vi "Logdata.vi"(7 "Command":T1, 8 "error in (no error)":errorcluster, 10 "Zone Setup Array":cluster{"Zone Selector":string, "Timing":dbl}[](array[cluster]), 11 "file path (dialog if empty)":path) -> (0 "error out":errorcluster, 2 "Zone Setup Array":cluster{"Zone Selector":string, "Timing":dbl}[](array[cluster]))   [LabVIEW 2013]
doc: "This subVi reads the data from Logdata.txt file and write all its value to the Zone Setup array in initialize state."
uses:
  Controls/Log data states.ctl
  <vilib>/Utility/file.llb/Write To Spreadsheet File (string).vi
  <vilib>/Utility/file.llb/Read From Spreadsheet File (string).vi
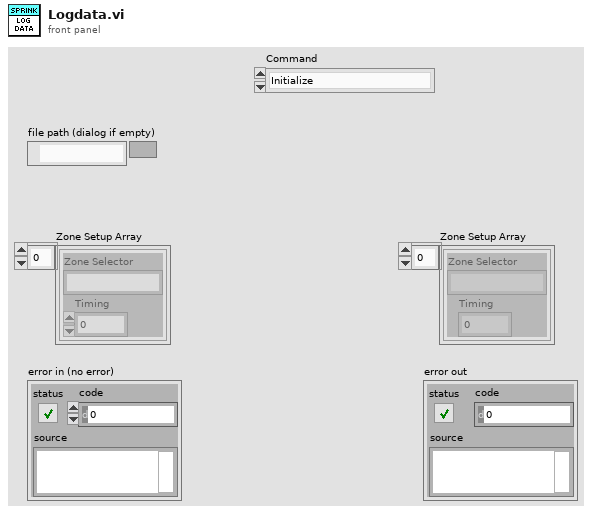
[diagram p1: front panel]
types:
  T1 = typedef "Log data states.ctl" = enum16{"Initialize", "Read", "Write", "Stop"}
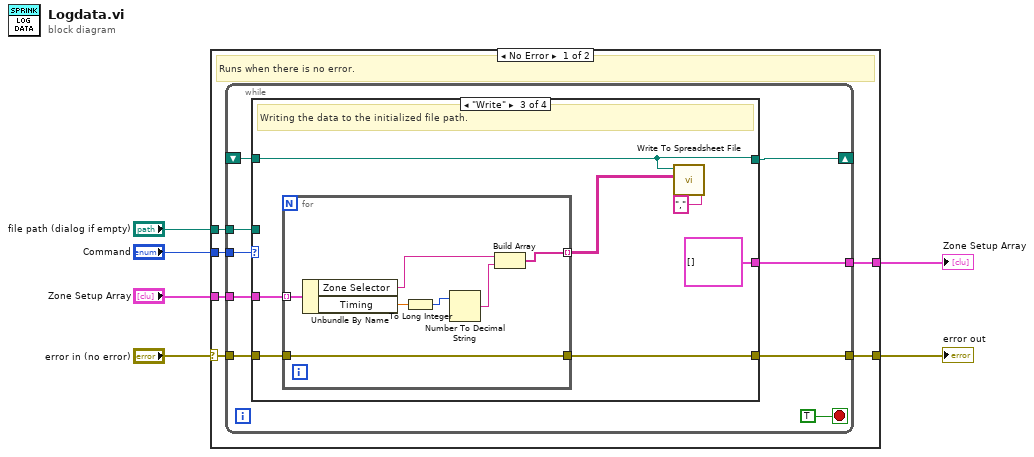
[diagram p0: block diagram]
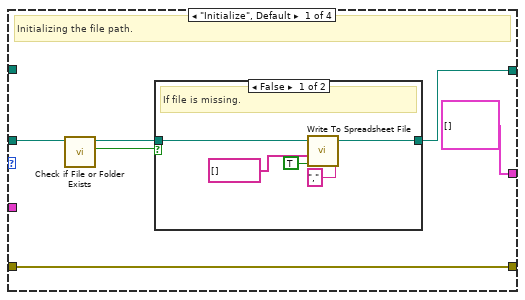
[diagram p2: hidden frame]
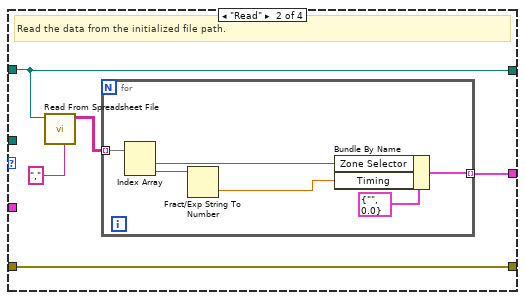
[diagram p4: hidden frame]
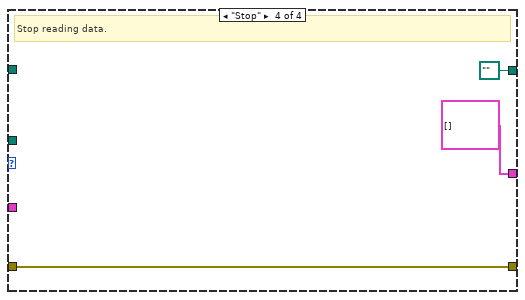
[diagram p5: hidden frame]
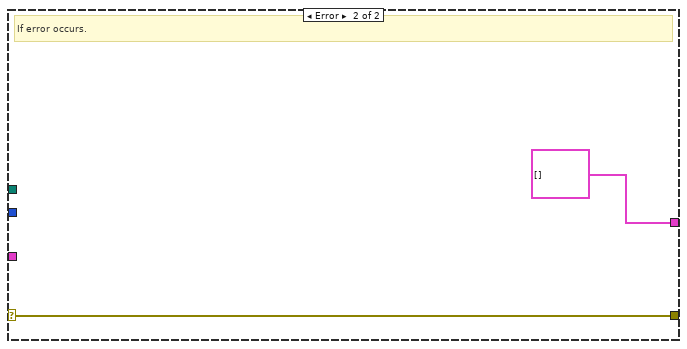
[diagram p6: hidden frame]
diagram:
  n1 = case shown="No Error" "error in (no error)" {
    selector: "error in (no error)" -> [w10 w63]
    tunnel: "file path (dialog if empty)" -> [w12 _]
    tunnel: "Command" -> [w11 _]
    tunnel: [w9 w63] -> w6
    tunnel: [w8 cluster{"Zone Selector":string, "Timing":dbl}[] []] -> w3
    tunnel: "Zone Setup Array" -> [w7 _]
    frame No Error {
      # "Runs when there is no error."
      n2 = while {
        tunnel: w12 -> [w19]
        shift-right: [w20] -> _
        shift-left: _ -> [w18]
        tunnel: w11 -> [w21]
        tunnel: w10 -> [w17]
        tunnel: [w16] -> w9
        tunnel: [w14] -> w8
        tunnel: w7 -> [w13]
        stop <- TRUE stop-if-true
        n3 = case shown="\"Write\"" w21 {
          tunnel: [w24 w34 w51 path "" ("new file path (Not A Path if cancelled)")] -> w20
          tunnel: w19 -> [w27 _ _ _]
          tunnel: w18 -> [_ w34 w51 _]
          tunnel: w17 -> [w23 w38 w46 w60]
          tunnel: [w23 w38 w47 w60] -> w16
          tunnel: [cluster{"Zone Selector":string, "Timing":dbl}[] [] w35 cluster{"Zone Selector":string, "Timing":dbl}[] [] cluster{"Zone Selector":string, "Timing":dbl}[] []] -> w14
          tunnel: w13 -> [_ _ w49 _]
          frame "Initialize", Default {
            # "Initializing the file path."
            n4 = call <vilib>:"Check if File or Folder Exists.vi"("path"=w27) -> ("file or folder exists?"=w26:bool, "dup path"=w25:path)  [unwired: 8 in, 1 out]
            n5 = case shown="False" w26 {
              tunnel: w25 -> [w32 w33]
              tunnel: [w31 w33] -> w24
              frame False {
                # "If file is missing."
                n6 = call-poly <vilib>:"Write To Spreadsheet File.vi"("delimiter (\\t)"="," ("delimiter (\\t)"), "append to file? (new file:F)"=TRUE, "1D data"=string[] [], "file path (dialog if empty)"=w32) -> ("new file path (Not A Path if cancelled)"=w31:path)  [unwired: 4 in]
              }
              frame True {
                # "Passing reference if file is there"
              }
            }
          }
          frame "Read" {
            # "Read the data from the initialized file path."
            n7 = call-poly <vilib>:"Read From Spreadsheet File.vi"("delimiter (\\t)"="," ("delimiter (\\t)"), "file path (dialog if empty)"=w34) -> ("all rows"=w36:string[][])  [unwired: 5 in, 4 out]
            n8 = for {
              tunnel: w36 -> [w44] mode=indexing
              tunnel: [w43] -> w35 mode=indexing
              n9 = Index Array(array=w44) -> (element #1=w40:string, element #2=w41:string)  [unwired: 2 in]
              n10 = Fract/Exp String To Number(string=w41) -> (number=w39:dbl)  [unwired: 3 in, 1 out]
              n11 = Bundle By Name(cluster=cluster{"Zone Selector":string, "Timing":dbl} {"Zone Selector"="", "Timing"=0.0} ("Zone Selector"), "Zone Selector"=w40, "Timing"=w39) -> (w43:cluster{"Zone Selector":string, "Timing":dbl})
            }
          }
          frame "Write" {
            # "Writing the data to the initialized file path."
            n12 = for {
              tunnel: w49 -> [w58] mode=indexing
              tunnel: [w56] -> w48 mode=indexing
              tunnel: [w55] -> w47
              tunnel: w46 -> [w55]
              n13 = Unbundle By Name(w58) -> ("Zone Selector"=w57:string, "Timing"=w54:dbl)
              n14 = To Long Integer(number=w54) -> (32bit integer=w52:i32)
              n15 = Number To Decimal String(number=w52) -> (decimal integer string=w53:string)  [unwired: 1 in]
              n16 = Build Array(w57, w53) -> (w56:string[])
            }
            n17 = call-poly <vilib>:"Write To Spreadsheet File.vi"("delimiter (\\t)"="," ("delimiter (\\t)"), "2D data"=w48, "file path (dialog if empty)"=w51) -> ()  [unwired: 5 in, 1 out]
          }
          frame "Stop" {
            # "Stop reading data."
          }
        }
      }
    }
    frame Error {
      # "If error occurs."
    }
  }
  "error out" <- w6
  "Zone Setup Array" <- w3
